vi "Internal Read.vi"(8 "error in (no error)":errorcluster, 10 "timeout ms":i32, 11 "WebSocket in":refnum<class "WebSocket.lvclass">) -> (0 "error out":errorcluster, 1 "Opcode":T1 items=["Cont. Frame"=0, "Text"=1, "Binary"=2, "Close Frame"=8, "Ping"=9, "Pong"=10], 2 "Data":u8[](array[numeric]), 3 "WebSocket out":refnum<class "WebSocket.lvclass">)   [LabVIEW 2013, in "WebSockets.lvlib" / "WebSocket.lvclass"]
doc: "Performs a read operation and handles internal WebSockets considerations.\n\n- Will read multi-framed messages as a single read\n- Automatically responds to Ping requests\n- Generates an error on receipt of a close frame\n\nVI will return when a 'complete' frame is read or a timeout occurs."
uses:
  WebSocket.lvclass
  Opcodes.ctl
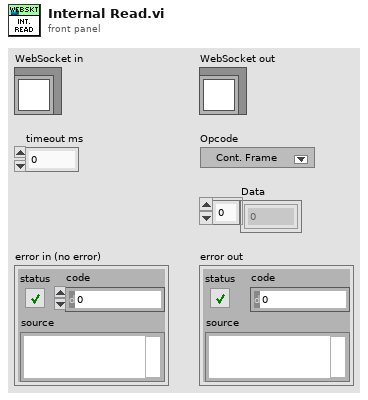
[diagram p1: front panel]
types:
  T1 = typedef "WebSockets.lvlib/WebSocket.lvclass/Opcodes.ctl" = u8
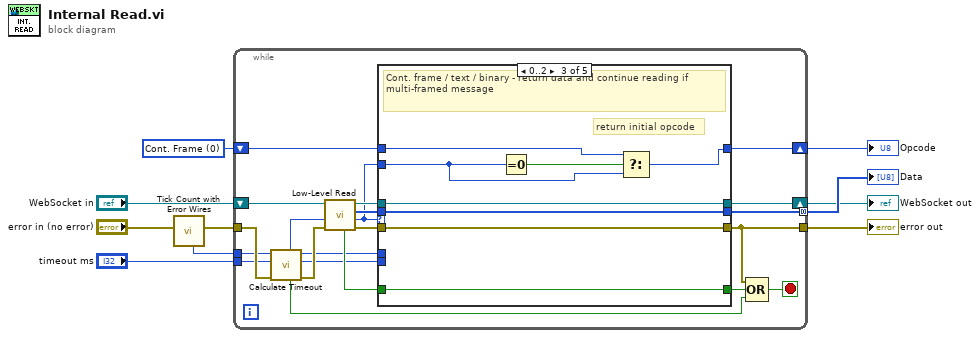
[diagram p0: block diagram]
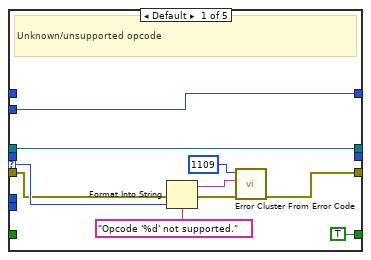
[diagram p2: hidden frame]
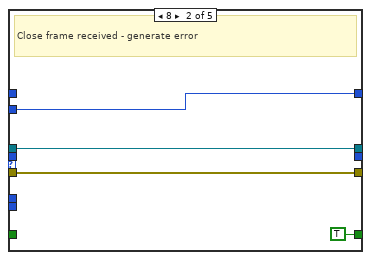
[diagram p3: hidden frame]
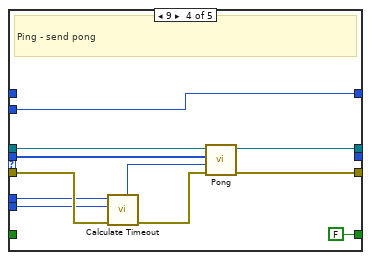
[diagram p4: hidden frame]
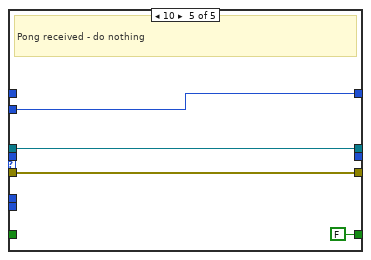
[diagram p5: hidden frame]
diagram:
  w1 = T1 0 items=["Cont. Frame"=0, "Text"=1, "Binary"=2, "Close Frame"=8, "Ping"=9, "Pong"=10] ("Opcode")
  n1 = call "Tick Count with Error Wires.vi"("error in (no error)"="error in (no error)") -> ("error out"=w3:errorcluster, "millisecond timer value"=w2:u32)  [unwired: 9 in]
  n2 = while {
    tunnel: w3 -> [w16]
    tunnel: "timeout ms" -> [w12]
    tunnel: [w26] -> w8
    shift-right: [w23] -> w7
    shift-left: "WebSocket in" -> [w29]
    tunnel: [w22] -> w10 mode=concatenating
    shift-right: [w19] -> w9
    shift-left: w1 -> [w17]
    tunnel: w2 -> [w13]
    stop <- w28 stop-if-true
    n3 = call "Calculate Timeout.vi"("error in (no error)"=w16, "timeout ms"=w12, "t0"=w13) -> ("error out"=w15:errorcluster, "Elapsed?"=w11:bool, "new timeout ms"=w14:i32)  [unwired: 6 in]
    n4 = call "Low-Level Read.vi"("error in (no error)"=w15, "timeout ms (5000)"=w14, "WebSockets in"=w29) -> ("error out"=w27:errorcluster, "Opcode"=w18:T1, "Data"=w24:u8[], "WebSockets out"=w25:refnum<class "WebSocket.lvclass">, "Finished?"=w20:bool)  [unwired: 4 in]
    n5 = case shown="0..2" w18 {
      selector: w18 -> [w34 _ _ _ _]
      tunnel: w27 -> [w33 w42 w50 w56 w65]
      tunnel: [w32 w42 w50 w60 w65] -> w26
      tunnel: w25 -> [w31 w41 w51 w62 w66]
      tunnel: w24 -> [_ _ w49 w61 _]
      tunnel: [w31 w41 w51 w59 w66] -> w23
      tunnel: [_ _ w49 _ _] -> w22
      tunnel: [TRUE ("Finished?") TRUE ("Finished?") w48 FALSE FALSE ("Finished?")] -> w21
      tunnel: w20 -> [_ _ w48 _ _]
      tunnel: [w30 w40 w46 w57 w63] -> w19
      tunnel: w18 -> [w30 w40 w44 w57 w63]
      tunnel: w17 -> [_ _ w45 _ _]
      tunnel: w13 -> [_ _ _ w55 _]
      tunnel: w12 -> [_ _ _ w54 _]
      frame Default {
        # "Unknown/unsupported opcode"
        n6 = Format Into String(format string="Opcode '%d' not supported.", error in=w33, w34) -> (resulting string=w37:string, error out=w38:errorcluster)  [unwired: 1 in]
        n7 = call <vilib>:"Error Cluster From Error Code.vi"("error in (no error)"=w38, "error message (\"\")"=w37, "error code (0)"=1109) -> ("error out"=w32:errorcluster)  [unwired: 6 in]
      }
      frame 8 {
        # "Close frame received - generate error"
      }
      frame 0..2 {
        # "return initial opcode"
        # "Cont. frame / text / binary - return data and continue reading if multi-framed message"
        n8 = Equal To 0?(x=w44) -> (x = 0?=w47:bool)
        n9 = Select(t=w45, s=w47, f=w44) -> (s? t:f=w46:T1)
      }
      frame 9 {
        # "Ping - send pong"
        n10 = call "Calculate Timeout.vi"("error in (no error)"=w56, "timeout ms"=w54, "t0"=w55) -> ("error out"=w53:errorcluster, "new timeout ms"=w52:i32)  [unwired: 6 in, 1 out]
        n11 = call-dynamic "Pong.vi"("error in (no error)"=w53, "timeout ms (5000)"=w52, "Ping Payload"=w61, "WebSocket in"=w62) -> ("error out"=w60:errorcluster, "WebSocket out"=w59:refnum<class "WebSocket.lvclass">)  [unwired: 6 in]
      }
      frame 10 {
        # "Pong received - do nothing"
      }
    }
    n12 = Compound Arithmetic op=OR(w26, w21, w11) -> (w28:bool)
  }
  "Data" <- w10
  "Opcode" <- w9
  "error out" <- w8
  "WebSocket out" <- w7
